vi "Sort QControl Class Hierarchy.vi"(11 "Class List in":string[][](array[string])) -> (3 "Class List out":string[][](array[string]))   [LabVIEW 2023, in "QControl Creation Wizard.lvclass"]
doc: "<b> </b> <b> </b>\n©2016 Q Software Innovations, LLC (QSI)\nwritten by Quentin Alldredge\nproduced in LabVIEW 2015\n\nsupport@qsoftwareinnovations.com\nwww.qsoftwareinnovations.com\n\nAll rights reserved.\n\nRedistribution and use in source and binary forms, with or without modification, are permitted provided that the following conditions are met:\n\n * Redistributions of source code must retain the above copyright notice, this list of conditions and the following disclaimer.\n * Redistributions in binary form must reproduce the above copyright notice, this list of conditions and the following disclaimer in the documentation and/or other materials provided with the distribution.\n * Neither the name of Q Software Innovations, LLC. nor the names of its contributors may be used to endorse or promote products derived from this software without specific prior written permission.\n\nTHIS SOFTWARE IS PROVIDED BY THE COPYRIGHT HOLDERS AND CONTRIBUTORS \"AS IS\" AND ANY EXPRESS OR IMPLIED WARRANTIES, INCLUDING, BUT NOT LIMITED TO, THE IMPLIED WARRANTIES OF MERCHANTABILITY AND FITNESS FOR A PARTICULAR PURPOSE ARE DISCLAIMED. IN NO EVENT SHALL THE COPYRIGHT OWNER OR CONTRIBUTORS BE LIABLE FOR ANY DIRECT, INDIRECT, INCIDENTAL, SPECIAL, EXEMPLARY, OR CONSEQUENTIAL DAMAGES (INCLUDING, BUT NOT LIMITED TO, PROCUREMENT OF SUBSTITUTE GOODS OR SERVICES; LOSS OF USE, DATA, OR PROFITS; OR BUSINESS INTERRUPTION) HOWEVER CAUSED AND ON ANY THEORY OF LIABILITY, WHETHER IN CONTRACT, STRICT LIABILITY, OR TORT (INCLUDING NEGLIGENCE OR OTHERWISE) ARISING IN ANY WAY OUT OF THE USE OF THIS SOFTWARE, EVEN IF ADVISED OF THE POSSIBILITY OF SUCH DAMAGE."
uses:
  QControl Creation Wizard.lvclass
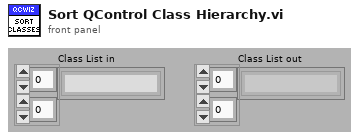
[diagram p1: front panel]
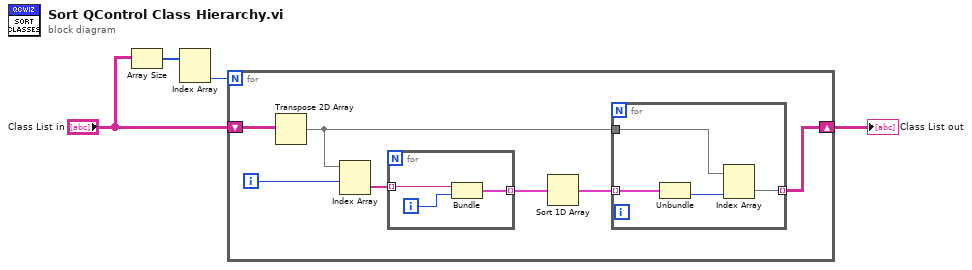
[diagram p0: block diagram]
diagram:
  n1 = Array Size(array="Class List in") -> (size(s)=w3:i32[])
  n2 = Index Array(array=w3) -> (element #2=w1:i32)  [unwired: 2 in, 1 out]
  n3 = for {
    N: w1 -> [_]
    shift-right: [w10] -> w4
    shift-left: "Class List in" -> [w9]
    i -> [w5]
    n4 = Transpose 2D Array(2D array=w9) -> (transposed array=w11:string[][])
    n5 = Index Array(array=w11, index (row)=w5) -> (element=w8:string[])  [unwired: 1 in]
    n6 = for {
      tunnel: w8 -> [w14] mode=indexing
      tunnel: [w12] -> w7 mode=indexing
      i -> [w13]
      n7 = Bundle("String"=w14, w13) -> (w12:cluster{"String":string, i32})  [unwired: 1 in]
    }
    n8 = Sort 1D Array(array=w7) -> (sorted array=w6:cluster{"String":string, i32}[])
    n9 = for {
      tunnel: w6 -> [w18] mode=indexing
      tunnel: w11 -> [w17]
      tunnel: [w16] -> w10 mode=indexing
      n10 = Unbundle(w18) -> (w15:i32)  [unwired: 1 out]
      n11 = Index Array(array=w17, index (col)=w15) -> (element=w16:string[])  [unwired: 1 in]
    }
  }
  "Class List out" <- w4
